vi "kvCanReadTimer.vi"(0 "Channel Handle (input only)":i32, 1 "error in (no error)":errorcluster) -> (2 "Channel Handle (ouput only)":i32, 3 "Current Time":u32, 4 "error out":errorcluster)   [LabVIEW 2022 SP3]
doc: "Reads the current time from the clock used to timestamp the messages for the indicated circuit."
uses:
  canlib32.dll
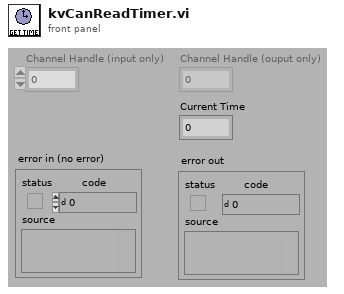
[diagram p1: front panel]
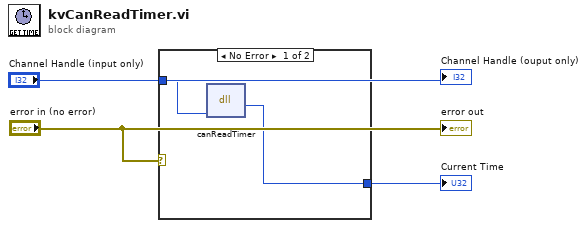
[diagram p0: block diagram]
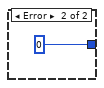
[diagram p2: hidden frame]
diagram:
  n1 = case shown="No Error" "error in (no error)" {
    tunnel: "Channel Handle (input only)" -> [w5 _]
    tunnel: [w4 0] -> w1
    frame No Error {
      n2 = dll-call lib="canlib32.dll" fn="canReadTimer" label="Call canReadTimer"("channelHandle"=w5) -> (w4:u32)  [unwired: 4 in, 2 out]
    }
    frame Error {
    }
  }
  "Current Time" <- w1
  "error out" <- "error in (no error)"
  "Channel Handle (ouput only)" <- "Channel Handle (input only)"
